vi "EjectCoin.vi"(8 "error in (no error)":errorcluster, 11 "GumballMachine in":refnum<class "GumballMachine.lvclass">) -> (0 "error out":errorcluster, 2 "ProcessMessage":string, 3 "GumballMachine out":refnum<class "GumballMachine.lvclass">)   [LabVIEW 2013, in "GumballMachine.lvclass"]
uses:
  GumballMachine.lvclass
  GumballMachine.lvclass/GumballMachine.ctl
  State.lvclass/State.lvclass
  StateMark.ctl
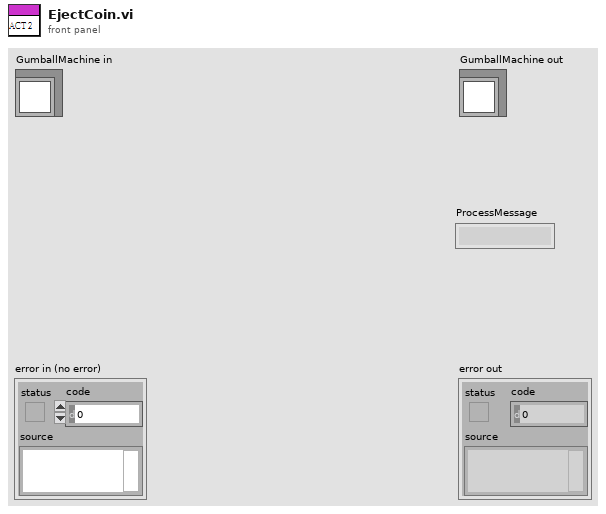
[diagram p1: front panel]
types:
  T1 = typedef "StateMark.ctl" = enum16{"沒有硬幣", "有硬幣", "賣出糖果", "糖果賣完", "NoChange"}
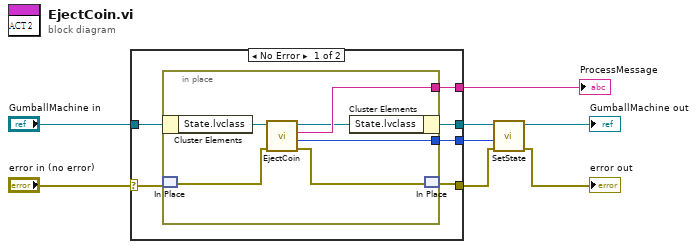
[diagram p0: block diagram]
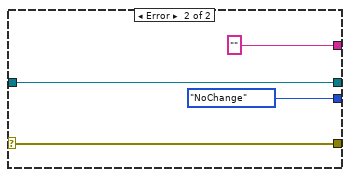
[diagram p2: hidden frame]
diagram:
  n1 = case shown="No Error" "error in (no error)" {
    selector: "error in (no error)" -> [w10 w24]
    tunnel: [w9 w24] -> w2
    tunnel: [w11 w23] -> w5
    tunnel: "GumballMachine in" -> [w13 w23]
    tunnel: [w14 "" ("ProcessMessage")] -> w6
    tunnel: [w12 StateMark."NoChange" ("NextState")] -> w3
    frame No Error {
      n2 = in-place {
        in-place-border: [w20] -> w14
        in-place-border: [w17] -> w12
        n3 = in-place-cluster #1(w13) -> ("State.lvclass"=w19:refnum<class "State.lvclass">)
        n4 = in-place-match #2(w10) -> (w15:errorcluster)
        n5 = call-dynamic "EjectCoin.vi"("error in (no error)"=w15, "State in"=w19) -> ("error out"=w16:errorcluster, "NextState"=w17:T1, "ProcessMessage"=w20:string, "State out"=w18:refnum<class "State.lvclass">)  [unwired: 6 in]
        n6 = in-place-cluster #1("State.lvclass"=w18) -> (w11:refnum<class "GumballMachine.lvclass">)
        n7 = in-place-match #2(w16) -> (w9:errorcluster)
      }
    }
    frame Error {
    }
  }
  "ProcessMessage" <- w6
  n8 = call-dynamic "SetState.vi"("error in (no error)"=w2, "State"=w3, "GumballMachine in"=w5) -> ("error out"=→"error out":errorcluster, "GumballMachine out"=→"GumballMachine out":refnum<class "GumballMachine.lvclass">)  [unwired: 7 in]
